vi "Switch Tables.vi"(0 "error in (no error)":errorcluster, 11 "Data.PG":refnum<class "LV-Data.PGSQL.lvclass">) -> (3 "Data.PG out":refnum<class "LV-Data.PGSQL.lvclass">, 8 "error out":errorcluster)   [LabVIEW 2016, in "LV-Data.PGSQL.lvclass"]
uses:
  LV-Data.PGSQL.lvclass
panel:
  in  "Columns to be Switched from old old Table":string[](array[string])
  in  "Number of Columns being moved":i32
  in  "Columns to be switch":string[][](array[string])
  in  "Existing Table":string
  in  "New Table":string
  out "SQL":string
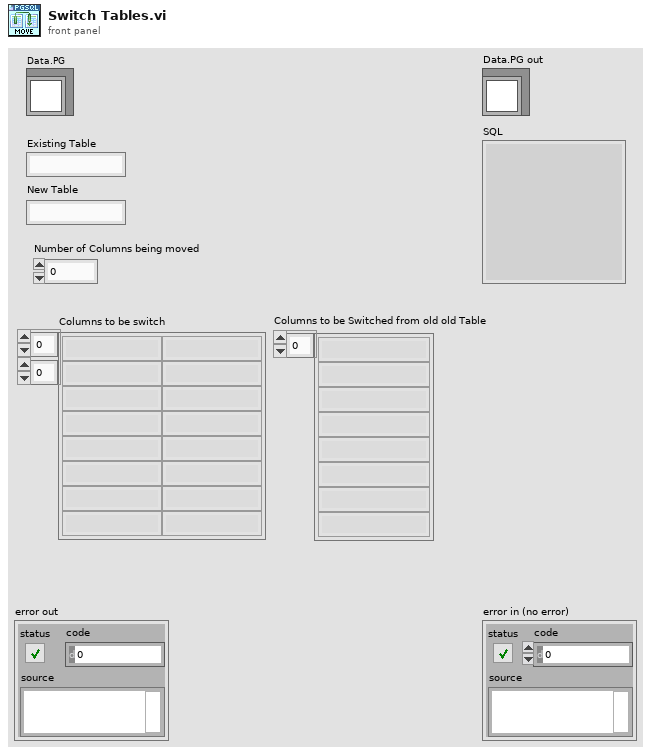
[diagram p1: front panel]
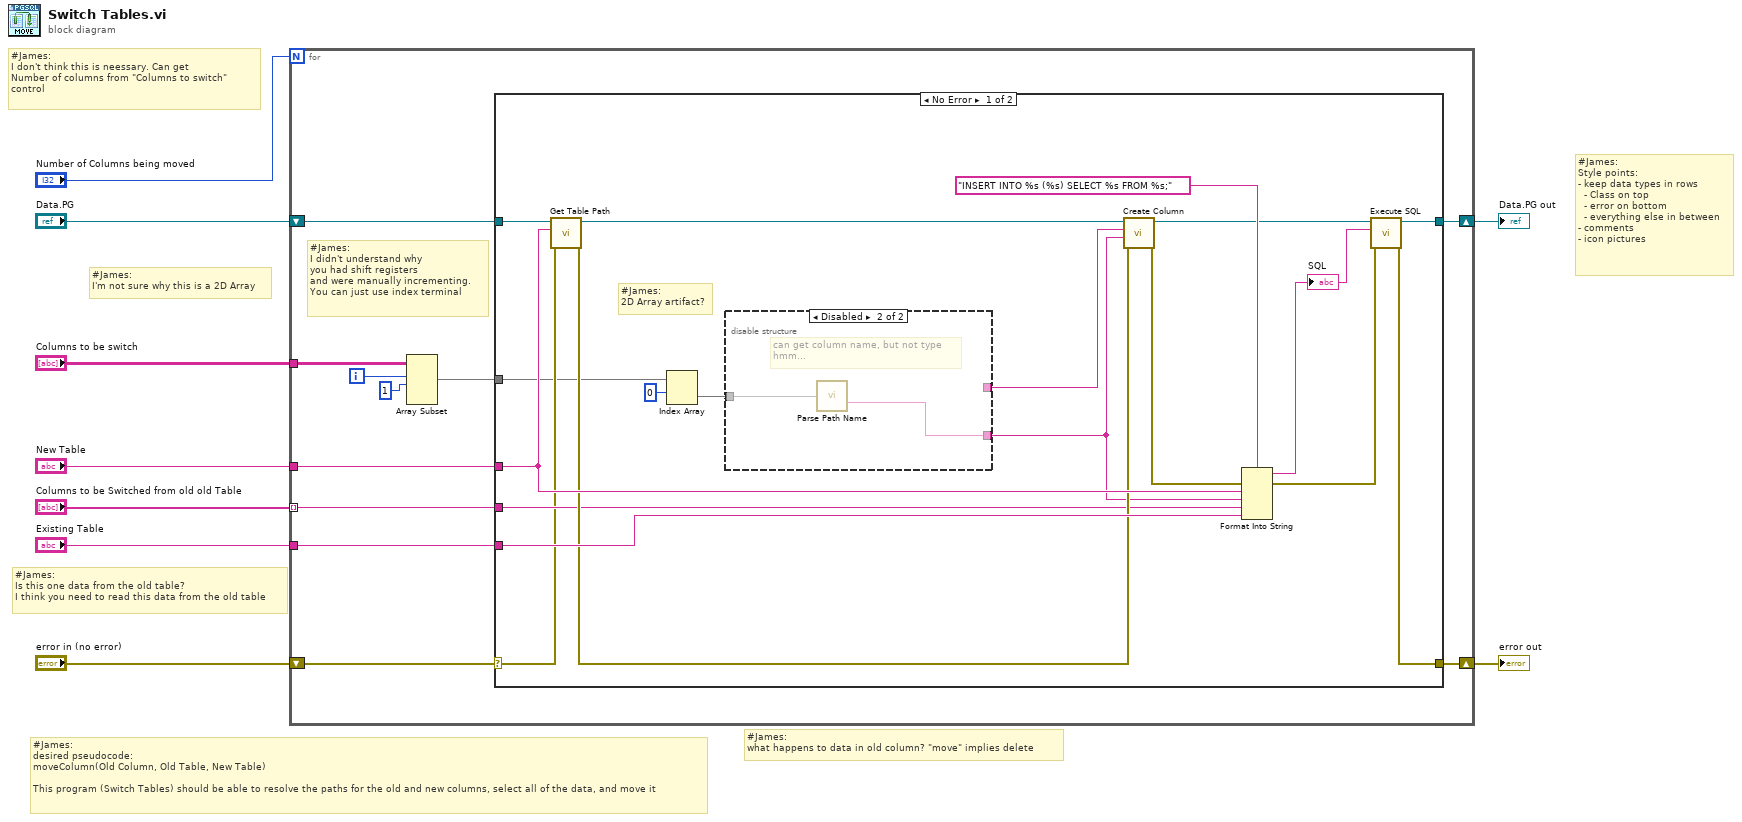
[diagram p0: block diagram]
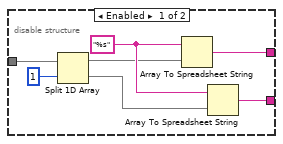
[diagram p2: hidden frame]
diagram:
  # "#James:\nwhat happens to data in old column? \"move\" implies delete"
  # "#James:\nStyle points:\n- keep data types in rows\n  - Class on top\n  - error on bottom\n  - everything else in between\n- comments\n- icon pictures"
  # "#James:\ndesired pseudocode:\nmoveColumn(Old Column, Old Table, New Table)\n\nThis program (Switch Tables) should be able to resolve the paths for the old and new columns, select all of the data, and move it"
  # "#James:\nIs this one data from the old table?\nI think you need to read this data from the old table"
  # "#James:\nI don't think this is neessary. Can get\nNumber of columns from \"Columns to switch\"\ncontrol"
  # "#James:\nI'm not sure why this is a 2D Array"
  n1 = for {
    N: "Number of Columns being moved" -> [_]
    tunnel: "New Table" -> [w20]
    tunnel: "Existing Table" -> [w19]
    tunnel: "Columns to be Switched from old old Table" -> [w15] mode=indexing
    shift-right: [w16] -> w5
    shift-left: "Data.PG" -> [w17]
    shift-right: [w18] -> w7
    shift-left: "error in (no error)" -> [w14]
    tunnel: "Columns to be switch" -> [w10]
    i -> [w12]
    # "#James:\nI didn't understand why\nyou had shift registers\nand were manually incrementing.\nYou can just use index terminal"
    n2 = Array Subset(array=w10, index (row)=w12, length (row)=1 ("length")) -> (w11:string[][])  [unwired: 2 in]
    n3 = case shown="No Error" w14 {
      selector: w14 -> [w30 w49]
      tunnel: w20 -> [w38 _]
      tunnel: w19 -> [w37 _]
      tunnel: [w35 w49] -> w18
      tunnel: w17 -> [w34 w50]
      tunnel: [w32 w50] -> w16
      tunnel: w15 -> [w31 _]
      tunnel: w11 -> [w23 _]
      frame No Error {
        # "#James:\n2D Array artifact?"
        n4 = call "Get Table Path.vi"("error in (no error)"=w30, "Table"=w38, "Data.PG"=w34) -> ("error out"=w36:errorcluster, "Data.PG out"=w33:refnum<class "LV-Data.PGSQL.lvclass">)  [unwired: 6 in, 1 out]
        n5 = Index Array(array=w23, index (row)=0) -> (element=w28:string[])  [unwired: 1 in]
        n6 = disable-structure shown="Disabled" {
          disable-tunnel: w28 -> [w46 w48]
          disable-tunnel: [w43 _] -> w26
          disable-tunnel: [w42 w47] -> w25
          frame Enabled {
            w45 = "%s" ("format string")
            n7 = Split 1D Array(array=w46, index=1) -> (first subarray=w41:string[], second subarray=w40:string[])
            n8 = Array To Spreadsheet String(array=w41, 3:w45) -> (spreadsheet string=w43:string)  [unwired: 1 in]
            n9 = Array To Spreadsheet String(array=w40, 3:w45) -> (spreadsheet string=w42:string)  [unwired: 1 in]
          }
          frame Disabled {
            # "can get column name, but not type\nhmm..."
            n10 = call "Parse Path Name.vi"("PG Path"=w48) -> ("Column name"=w47:string)  [unwired: 10 in, 4 out]
          }
        }
        n11 = call "Create Column.vi"("error in (no error)"=w36, "new column name"=w25, "new column data type"=w26, "Data.PGSQL in"=w33) -> ("error out"=w22:errorcluster, "Data.PGSQL out"=w24:refnum<class "LV-Data.PGSQL.lvclass">)  [unwired: 6 in]
        n12 = Format Into String(format string="INSERT INTO %s (%s) SELECT %s FROM %s;", error in=w22, w38, w25, w31, w37) -> (resulting string=w21:string, error out=w29:errorcluster)  [unwired: 1 in]
        "SQL" <- w21
        n13 = call "Execute SQL.vi"("error in"=w29, "SQL"=w21, "Data.PG"=w24) -> ("error out"=w35:errorcluster, "Data.PG out"=w32:refnum<class "LV-Data.PGSQL.lvclass">)  [unwired: 6 in, 1 out]
      }
      frame Error {
      }
    }
  }
  "error out" <- w7
  "Data.PG out" <- w5
